vi "SettingsArraytoINI.vi"(8 "error in (no error)":errorcluster, 10 "Settings Array IN":T1[](array[typedef]), 11 "Path":path) -> (0 "error out":errorcluster)   [LabVIEW 2012]
doc: "SciScan 1.2 160622\nThis VI reads an INI file and stores all keys in a Generalized Functional Global Variable (GFG). It then monitors updates to the GFG and writes keys back into INI file before closing. Note that the INI file only supports data type DBL or STRING. The GFG can handle any arbitrary data type, but values that are not DBL or STRING are discarded when closing and not written to INI file."
uses:
  Plugins/Macro Module/MacroGUI Module/Custom Controls and Typedefs/GFG Variable for IO.ctl
  <vilib>/Utility/config.llb/Write Key (Double).vi
  <vilib>/Utility/config.llb/Write Key (String).vi
  <vilib>/Utility/config.llb/Write Key (Boolean).vi
  <vilib>/Utility/config.llb/NI_LVConfig.lvlib
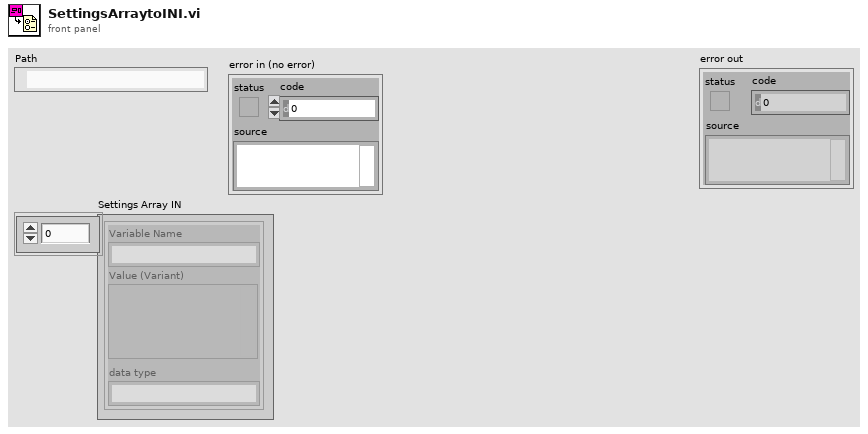
[diagram p1: front panel]
types:
  T1 = typedef "GFG Variable for IO.ctl" = cluster{"Variable Name":string, "Value (Variant)":variant, "data type":string}
  T2 = typedef "NI_LVConfig.lvlib/Config Data RefNum.ctl" = refnum<k1>
  T3 = typedef "VariantType.lvlib/Type.ctl" = enum8{"Invalid Type", "Void", "I8", "I16", "I32", "I64", "U8", "U16", "U32", "U64", "Single Float", "Double Float", "Extended Float", "Single Complex", "Double Complex", "Extended Complex", "Enum U8", "Enum U16", "Enum U32", "Enum U64", "Single Float With Unit", "Double Float With Unit", "Extended Float With Unit", "Single Complex with Unit", "Double Complex with Unit", "Extended Complex with Unit", "Boolean", "String", "Path", "Picture", "Tag", "Array", "Cluster", "Variant", "LV Variant", "Waveform", "Timestamp", "Digital Waveform", "Digital Data", "ExpressData", "Refnum", "External Data", "VI", "Poly VI", "LabVIEW Class Instance", "Fixed Point"}
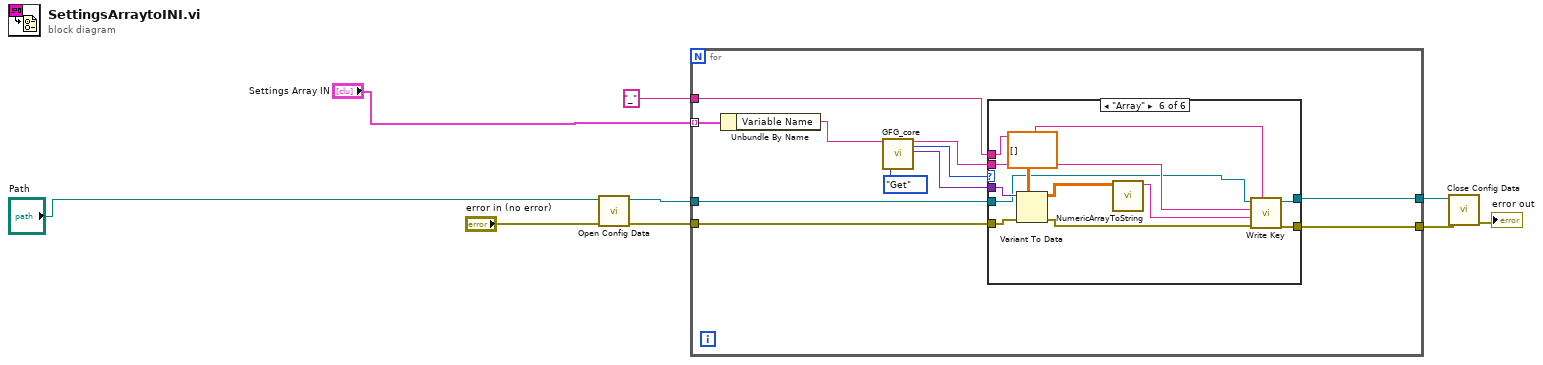
[diagram p0: block diagram]
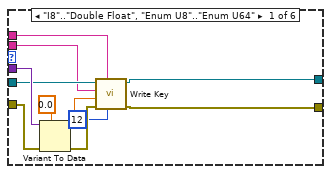
[diagram p2: hidden frame]
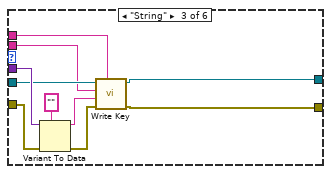
[diagram p4: hidden frame]
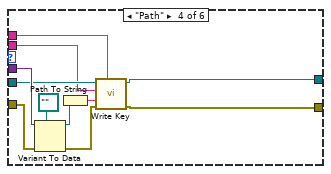
[diagram p5: hidden frame]
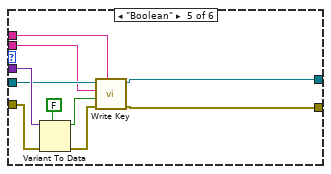
[diagram p6: hidden frame]
diagram:
  n1 = call <vilib>:"Open Config Data.vi"("error in (no error)"="error in (no error)", "configuration file path"="Path") -> ("error out"=w7:errorcluster, "refnum"=w8:T2)  [unwired: 7 in, 1 out]
  n2 = for {
    tunnel: [w19] -> w4
    tunnel: w8 -> [w18]
    tunnel: w7 -> [w20]
    tunnel: [w17] -> w5
    tunnel: "Settings Array IN" -> [w11] mode=indexing
    tunnel: "_" ("Variable Name") -> [w16]
    n3 = Unbundle By Name(w11) -> ("Variable Name"=w10:string)
    n4 = call "GFG_core.vi"("Variable Name in"=w10, "Action"=enum16{"Init", "Set", "Get"}."Get") -> ("Variable Name Out"=w12:string, "Data Type Out"=w14:T3, "Variant Out"=w13:variant)  [unwired: 11 in, 4 out]
    n5 = case shown="\"Array\"" w14 {
      tunnel: w13 -> [w30 _ w43 w54 w64 w75]
      tunnel: [w27 w33 w40 w52 w61 w71] -> w19
      tunnel: w20 -> [w26 w33 w39 w51 w60 w73]
      tunnel: w18 -> [w25 w32 w38 w50 w59 w67]
      tunnel: [w24 w32 w37 w49 w58 w66] -> w17
      tunnel: w12 -> [w23 _ w36 w48 w57 w68]
      tunnel: w16 -> [w22 _ w35 w47 w56 w65]
      frame "I8".."Double Float", "Enum U8".."Enum U64" {
        n6 = Variant To Data(error in=w26, type=0.0, Variant=w30) -> (data=w29:dbl, error out=w28:errorcluster)
        n7 = call-poly <vilib>:"Write Key.vi"("precision (6)"=i16 12, "section"=w22, "error in (no error)"=w28, "value"=w29, "key"=w23, "refnum"=w25) -> ("error out"=w27:errorcluster, "refnum out"=w24:T2)  [unwired: 3 in, 1 out]
      }
      frame Default {
      }
      frame "String" {
        n8 = Variant To Data(error in=w39, type="" ("Variable Name Out"), Variant=w43) -> (data=w42:string, error out=w41:errorcluster)
        n9 = call-poly <vilib>:"Write Key.vi"("section"=w35, "error in (no error)"=w41, "value"=w42, "key"=w36, "refnum"=w38) -> ("error out"=w40:errorcluster, "refnum out"=w37:T2)  [unwired: 4 in, 1 out]
      }
      frame "Path" {
        n10 = Variant To Data(error in=w51, type=path "" ("configuration file path 2"), Variant=w54) -> (data=w44:path, error out=w53:errorcluster)
        n11 = Path To String(path=w44) -> (string=w45:string)
        n12 = call-poly <vilib>:"Write Key.vi"("section"=w47, "error in (no error)"=w53, "value"=w45, "key"=w48, "refnum"=w50) -> ("error out"=w52:errorcluster, "refnum out"=w49:T2)  [unwired: 4 in, 1 out]
      }
      frame "Boolean" {
        n13 = Variant To Data(error in=w60, type=FALSE, Variant=w64) -> (data=w63:bool, error out=w62:errorcluster)
        n14 = call-poly <vilib>:"Write Key.vi"("section"=w56, "error in (no error)"=w62, "value"=w63, "key"=w57, "refnum"=w59) -> ("error out"=w61:errorcluster, "refnum out"=w58:T2)  [unwired: 4 in, 1 out]
      }
      frame "Array" {
        n15 = Variant To Data(error in=w73, type=dbl[][] [], Variant=w75) -> (data=w70:dbl[][], error out=w72:errorcluster)
        n16 = call "NumericArrayToString.vi"("Array In"=w70) -> ("String Out"=w69:string)  [unwired: 10 in]
        n17 = call-poly <vilib>:"Write Key.vi"("section"=w65, "error in (no error)"=w72, "value"=w69, "key"=w68, "refnum"=w67) -> ("error out"=w71:errorcluster, "refnum out"=w66:T2)  [unwired: 4 in, 1 out]
      }
    }
  }
  n18 = call <vilib>:"Close Config Data.vi"("error in (no error)"=w4, "refnum"=w5) -> ("error out"=→"error out":errorcluster)  [unwired: 8 in, 1 out]
